vi "Man_Booked_Details.vi"(8 "error in (no error)":errorcluster, 10 "Column":string[](array[string]), 11 "Refnum in":T1) -> (0 "error out":errorcluster, 2 "Data":string[](array[string]), 3 "Refnum Out":T1)   [LabVIEW 2020]
uses:
  <vilib>/addons/database/Connection.llb/Conn ObjectReference.ctl
  <userlib>/_OpenG.lib/array/array.llb/Remove Duplicates from 1D Array (String)__ogtk.vi
  <vilib>/addons/database/_DB Variant To Data/Database Variant To Data.xnode
  <vilib>/addons/database/NI_Database_API.lvlib
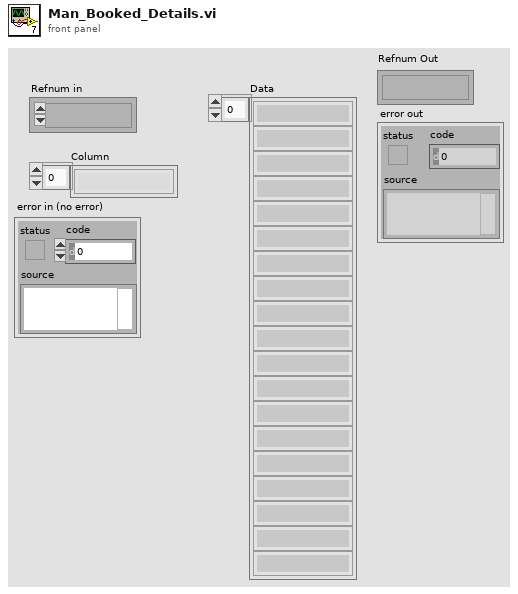
[diagram p1: front panel]
types:
  T1 = typedef "NI_Database_API.lvlib/Conn ObjectReference.ctl" = refnum<k1>
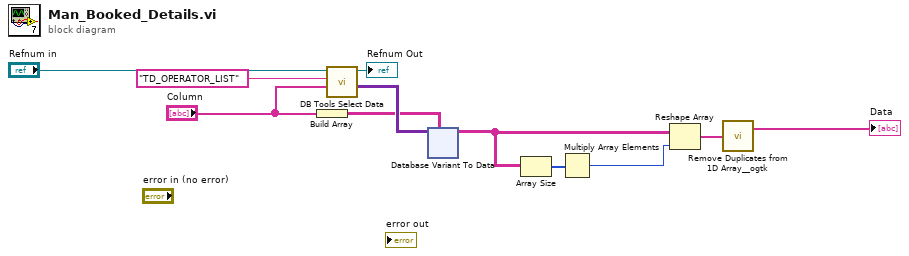
[diagram p0: block diagram]
diagram:
  n1 = Build Array("Column") -> (w2:string[][])
  n2 = call <vilib>:"DB Tools Select Data.vi"("columns"="Column", "table"="TD_OPERATOR_LIST", "connection reference"="Refnum in") -> ("data"=w4:variant[][], "connection reference out"=→"Refnum Out":T1)  [unwired: 3 in, 1 out]
  n3 = xnode "Database Variant To Data"("database variant"=w4, "type"=w2) -> ("data"=w8:string[][])  [unwired: 1 in, 1 out]
  n4 = Array Size(array=w8) -> (size(s)=w7:i32[])
  n5 = Multiply Array Elements(1:w7) -> (0:w9:i32)
  n6 = Reshape Array(w8, w9) -> (w10:string[])
  n7 = call-poly <userlib>:"Remove Duplicates from 1D Array__ogtk.vi"("Input Array"=w10) -> ("Output Array"=→"Data":string[])  [unwired: 1 out]
